vi "Teleop.vi"(10 "Match Info":T1={"Autonomous Elapsed Seconds"=0.0, "TeleOp Elapsed Seconds"=0.0, "Disabled Elapsed Seconds"=0.0, "Visited Autonomous"=FALSE, "Visited TeleOp"=FALSE, "Visited Disabled"=FALSE, "Autonomous Settings"={"Autonomous Style"=enum."Independent", "VI Refnum"=refnum}}, 11 "Call Context":T2) -> ()   [LabVIEW 2014]
doc: "This VI is called for each TeleOp packet received from the DS where the robot is not disabled. It is often used to read from the joysticks and update I/O or to update setpoints for timed control loops. It should complete and return within 20 milliseconds or it may miss DS packets."
uses:
  <vilib>/Rock Robotics/WPI/DriverStation/WPI_DriverStationDerivedRobotMode.ctl
  <vilib>/Rock Robotics/WPI/DriverStation/WPI_DriverStationMatch Info.ctl
  <vilib>/Rock Robotics/WPI/RobotDrive/WPI_RobotDriveGetSetRefNum.vi
  <vilib>/Rock Robotics/WPI/Joystick/WPI_JoystickGetSetRefNum.vi
  Robot Global Data.vi
  <vilib>/Rock Robotics/Network Tables/SD Write Boolean Array.vi
  <vilib>/Rock Robotics/Network Tables/SD Write Numeric Array.vi
  <vilib>/Rock Robotics/Network Tables/SD Read Boolean.vi
  <vilib>/Rock Robotics/Network Tables/SD Read Number.vi
  <vilib>/Rock Robotics/WPI/RobotDrive/WPI_RobotDriveArcadeDrive_Standard(NoSaturation).vi
panel:
  out "Sample Slider 0":dbl(slide) scale=0.0..5.0
  out "Sample Boolean 1":bool
  out "Sample Boolean 0":bool
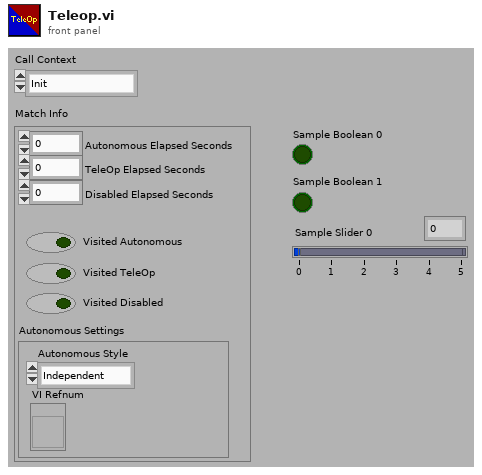
[diagram p1: front panel]
types:
  T1 = typedef "WPI_DriverStationMatch Info.ctl" = cluster{"Autonomous Elapsed Seconds":dbl, "TeleOp Elapsed Seconds":dbl, "Disabled Elapsed Seconds":dbl, "Visited Autonomous":bool, "Visited TeleOp":bool, "Visited Disabled":bool, "Autonomous Settings":cluster{"Autonomous Style":enum16{"Iterative", "Independent"}, "VI Refnum":refnum<vi>}}
  T2 = typedef "WPI_DriverStationDerivedRobotMode.ctl" = enum16{"Init", "Execute", "Stop"}
  T3 = typedef "WPI_RobotDriveDevRef.ctl" = cluster{"DevStatus":errorcluster, "Motors[]":T4[], "Square Inputs":bool, "Max Output":dbl}
  T4 = typedef "WPI_MotorControlDeviceRef.ctl" = cluster{"DeviceStatus":errorcluster, "Type":T5, "PWM":cluster{"Controller":T6, "PWM Channel":T7, "DeadBand":T8}, "CAN":cluster{"Device Number":u8, "Control Mode":T9, "Semaphore":T10, "Max Vout":dbl, "TalonSRX Control Mode":T11}, "Invert":bool, "TransformRef":T12, "InvTransformRef":T12}
  T5 = typedef "WPI_MotorControlType.ctl" = enum16{"PWM", "CAN", "CANTalonSRX"}
  T6 = typedef "FPGA_TypedefDigitalModule.ctl" = enum16{"Controller 1"}
  T7 = typedef "FPGA_DIOPWMChannel.ctl" = enum8{"PWM 0", "PWM 1", "PWM 2", "PWM 3", "PWM 4", "PWM 5", "PWM 6", "PWM 7", "PWM 8", "PWM 9", "PWM MXP 0", "PWM MXP 1", "PWM MXP 2", "PWM MXP 3", "PWM MXP 4", "PWM MXP 5", "PWM MXP 6", "PWM MXP 7", "PWM MXP 8", "PWM MXP 9", "Invalid"}
  T8 = typedef "WPI_PWMDeadband.ctl" = cluster{"Name":string, "maxPositivePwm":i32, "minPositivePwm":i32, "centerPwm":i32, "maxNegativePwm":i32, "minNegativePwm":i32, "angularRange":u16}
  T9 = typedef "WPI_CANJaguar_ControlMode.ctl" = enum8{"Percent VBus", "Current", "Speed", "Position", "Voltage"}
  T10 = typedef "Semaphore RefNum" = refnum<k1>
  T11 = typedef "WPI_CANTalonSRX_APIControlMode.ctl" = enum8{"Percent VBus", "Speed", "Position", "Slave", "Unchanged / Invalid"}
  T12 = typedef "WPI_PWMTransform_ConPane.ctl" = refnum<vi>
  T13 = typedef "WPI_JoystickDevRef.ctl" = cluster{"Device":T14}
  T14 = typedef "WPI_JoystickDeviceEnum.ctl" = enum16{"USB 0", "USB 1", "USB 2", "USB 3", "USB 4", "USB 5"}
  T15 = cluster{"Buttons[0]":bool, "Buttons[1]":bool, "Buttons[2]":bool, "Buttons[3]":bool, "Buttons[4]":bool, "Buttons[5]":bool, "Buttons[6]":bool, "Buttons[7]":bool, "Buttons[8]":bool}
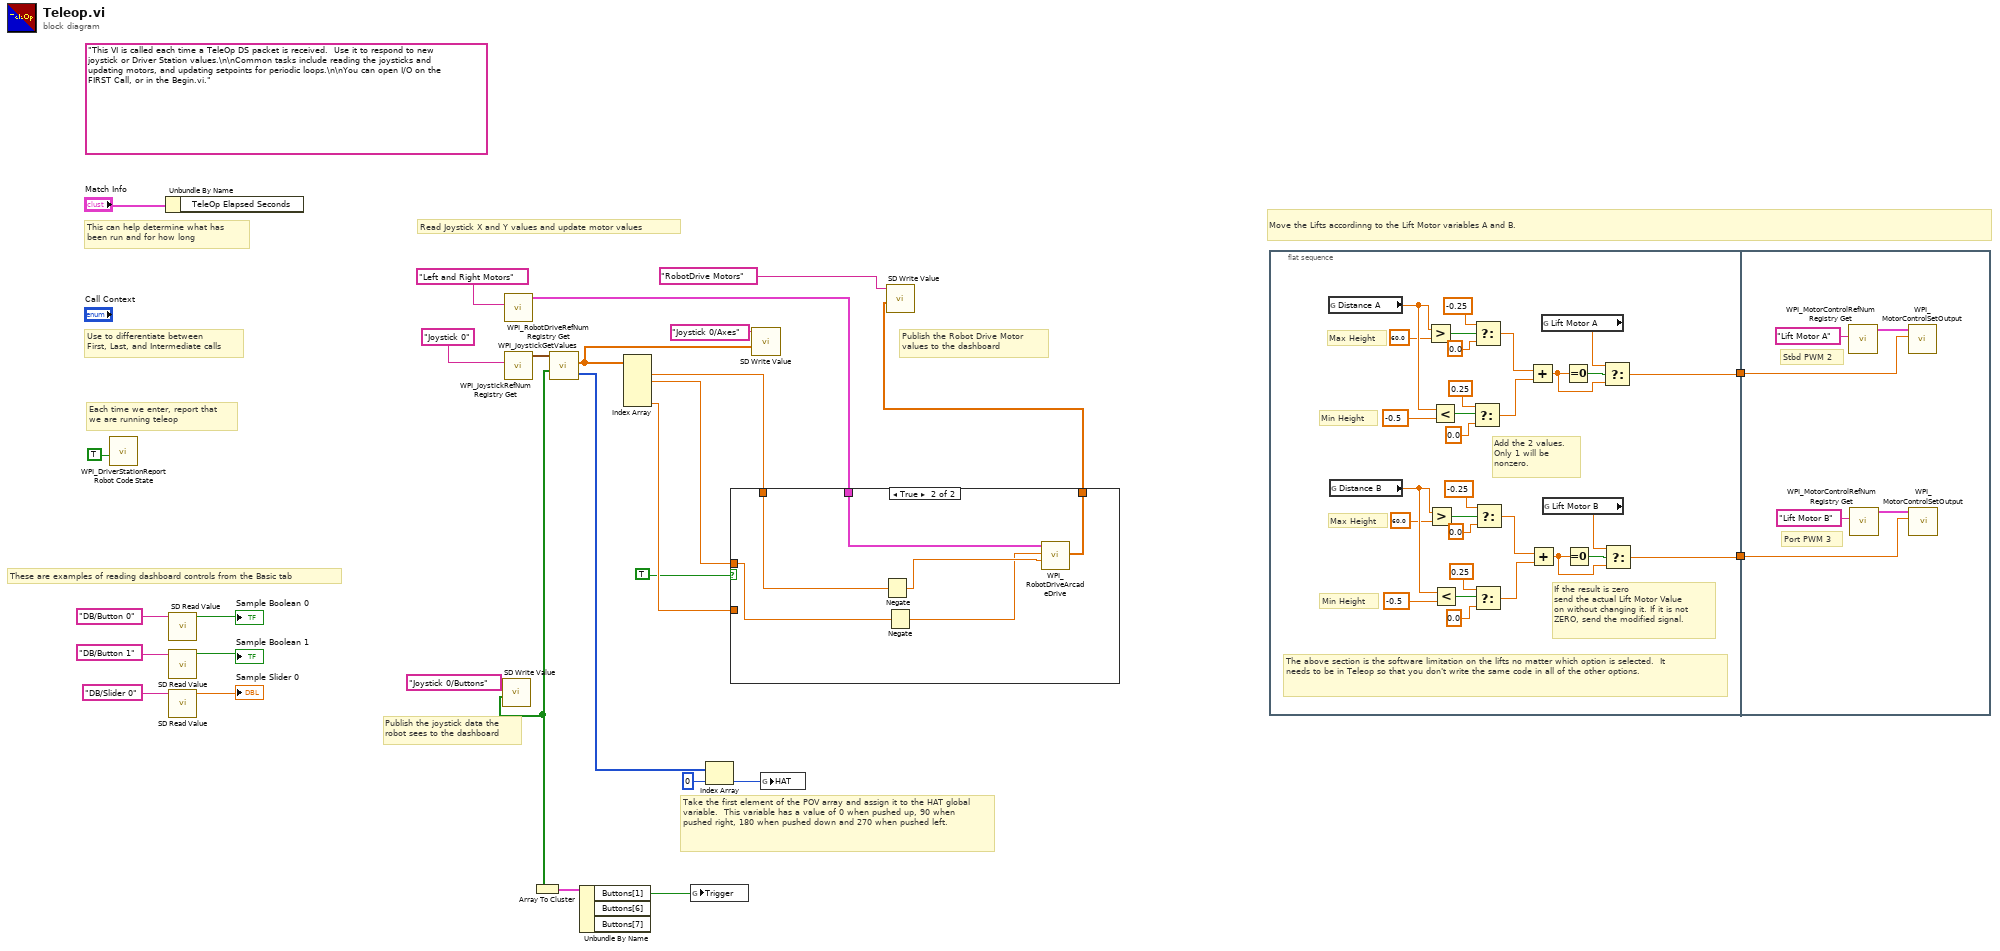
[diagram p0: block diagram]
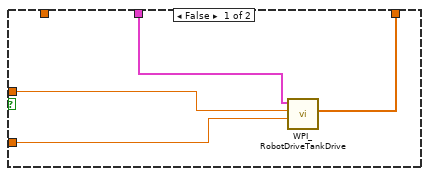
[diagram p2: hidden frame]
diagram:
  (unwired) "This VI is called each time a TeleOp DS packet is received.  Use it to respond to new joystick or Driver Station values.\n\nCommon tasks include reading the joysticks and updating motors, and updating setpoints for periodic loops.\n\nYou can open I/O on the FIRST Call, or in the Begin.vi."
  # "Move the Lifts accordinng to the Lift Motor variables A and B."
  # "Take the first element of the POV array and assign it to the HAT global variable.  This variable has a value of 0 when pushed up, 90 when pushed right, 180 when pushed down and 270 when pushed left."
  # "These are examples of reading dashboard controls from the Basic tab"
  # "Publish the Robot Drive Motor\nvalues to the dashboard"
  # "Publish the joystick data the\nrobot sees to the dashboard"
  # "Each time we enter, report that\nwe are running teleop"
  # "Use to differentiate between\nFirst, Last, and Intermediate calls"
  # "This can help determine what has\nbeen run and for how long"
  # "Read Joystick X and Y values and update motor values"
  n1 = call <vilib>:"WPI_DriverStationReport Robot Code State.vi"("TeleOp"=TRUE ("Autonomous")) -> ()  [unwired: 10 in, 1 out]
  n2 = Unbundle By Name("Match Info") -> ()  [unwired: 1 out]
  n3 = call-poly <vilib>:"SD Read Value.vi"("Name"="DB/Button 0" ("refnum name")) -> ("Boolean"=→"Sample Boolean 0":bool)  [unwired: 8 in, 2 out]
  n4 = call-poly <vilib>:"SD Read Value.vi"("Name"="DB/Button 1" ("refnum name")) -> ("Boolean"=→"Sample Boolean 1":bool)  [unwired: 8 in, 2 out]
  n5 = call-poly <vilib>:"SD Read Value.vi"("Name"="DB/Slider 0" ("refnum name")) -> ("Numeric"=→"Sample Slider 0":dbl)  [unwired: 8 in, 2 out]
  n6 = call <vilib>:"WPI_RobotDriveRefNum Registry Get.vi"("refnum name"="Left and Right Motors") -> ("RobotDriveDevRef"=w14:T3)  [unwired: 1 in, 9 out]
  n7 = call <vilib>:"WPI_JoystickRefNum Registry Get.vi"("refnum name"="Joystick 0") -> ("JoystickDevRef"=w26:T13)  [unwired: 1 in, 9 out]
  n8 = call <vilib>:"WPI_JoystickGetValues.vi"("JoystickDevRef"=w26) -> ("Buttons"=w13:bool[], "Axes"=w8:dbl[], "POVs"=w6:i16[])  [unwired: 6 in, 2 out]
  n9 = call-poly <vilib>:"SD Write Value.vi"("Boolean Array"=w13, "Name"="Joystick 0/Buttons") -> ()  [unwired: 8 in, 2 out]
  n10 = Array To Cluster(array=w13) -> (cluster=w12:T15)
  n11 = Unbundle By Name(w12) -> ("Buttons[1]"=w7:bool)  [unwired: 2 out]
  n12 = Index Array(array=w8) -> (element #1=w11:dbl, element #2=w10:dbl, element #5=w9:dbl)  [unwired: 5 in, 2 out]
  n13 = global write "Robot Global Data.vi" "Trigger"(w7) -> ()
  n14 = Index Array(array=w6, index=0) -> (element=w4:i16)
  n15 = case shown="True" TRUE {
    tunnel: [w33 w39] -> w15
    tunnel: w14 -> [w32 w38]
    tunnel: w11 -> [_ w37]
    tunnel: w10 -> [w31 w35]
    tunnel: w9 -> [w30 _]
    frame False {
      n16 = call <vilib>:"WPI_RobotDriveTankDrive.vi"("Right axis value"=w30, "Left axis value"=w31, "RobotDriveDevRef"=w32) -> ("Motor Values"=w33:dbl[])  [unwired: 6 in, 2 out]
    }
    frame True {
      n17 = Negate(x=w37) -> (-x=w36:dbl)
      n18 = Negate(x=w35) -> (-x=w34:dbl)
      n19 = call-poly <vilib>:"WPI_RobotDriveArcadeDrive.vi"("Y axis value"=w36, "X axis value"=w34, "RobotDriveDevRef"=w38) -> ("Motor Values"=w39:dbl[])  [unwired: 6 in, 2 out]
    }
  }
  n20 = call-poly <vilib>:"SD Write Value.vi"("Numeric Array"=w8, "Name"="Joystick 0/Axes") -> ()  [unwired: 8 in, 2 out]
  n21 = global write "Robot Global Data.vi" "HAT"(w4) -> ()
  n22 = call-poly <vilib>:"SD Write Value.vi"("Numeric Array"=w15, "Name"="RobotDrive Motors") -> ()  [unwired: 8 in, 2 out]
  n23 = flat-sequence {
    tunnel: [w41] -> w2
    tunnel: [w40] -> w1
    tunnel: w2 -> [w71]
    tunnel: w1 -> [w70]
    frame #0 {
      # "If the result is zero\nsend the actual Lift Motor Value\non without changing it. If it is not\nZERO, send the modified signal."
      # "Min Height"
      # "Max Height"
      # "Min Height"
      # "Max Height"
      # "The above section is the software limitation on the lifts no matter which option is selected.  It needs to be in Teleop so that you don't write the same code in all of the other options."
      # "Add the 2 values.  Only 1 will be nonzero."
      n24 = global read "Robot Global Data.vi" "Distance A"() -> (w61:dbl)
      n25 = global read "Robot Global Data.vi" "Distance B"() -> (w47:dbl)
      n26 = Greater?(x=w61, y=60.0) -> (0:w60:bool)
      n27 = Greater?(x=w47, y=60.0) -> (0:w46:bool)
      n28 = Less?(x=w61, y=-0.5) -> (x < y?=w63:bool)
      n29 = Less?(x=w47, y=-0.5) -> (x < y?=w49:bool)
      n30 = Select(t=0.25, s=w63, f=0.0) -> (s? t:f=w69:dbl)
      n31 = Select(t=-0.25, s=w60, f=0.0) -> (s? t:f=w68:dbl)
      n32 = Select(t=0.25, s=w49, f=0.0) -> (s? t:f=w55:dbl)
      n33 = Select(t=-0.25, s=w46, f=0.0) -> (s? t:f=w54:dbl)
      n34 = Add(x=w68, y=w69) -> (x+y=w56:dbl)
      n35 = Add(x=w54, y=w55) -> (x+y=w42:dbl)
      n36 = global read "Robot Global Data.vi" "Lift Motor A"() -> (w57:dbl)
      n37 = global read "Robot Global Data.vi" "Lift Motor B"() -> (w43:dbl)
      n38 = Equal To 0?(x=w56) -> (x = 0?=w58:bool)
      n39 = Equal To 0?(x=w42) -> (x = 0?=w44:bool)
      n40 = Select(t=w57, s=w58, f=w56) -> (s? t:f=w40:dbl)
      n41 = Select(t=w43, s=w44, f=w42) -> (s? t:f=w41:dbl)
    }
    frame #1 {
      # "Stbd PWM 2"
      # "Port PWM 3"
      n42 = call <vilib>:"WPI_MotorControlRefNum Registry Get.vi"("refnum name"="Lift Motor A") -> ("MotorControlDevRef"=w73:T4)  [unwired: 9 in, 1 out]
      n43 = call <vilib>:"WPI_MotorControlRefNum Registry Get.vi"("refnum name"="Lift Motor B") -> ("MotorControlDevRef"=w75:T4)  [unwired: 9 in, 1 out]
      n44 = call <vilib>:"WPI_MotorControlSetOutput.vi"("Output"=w70, "MotorControlDevRef"=w73) -> ()  [unwired: 7 in, 3 out]
      n45 = call <vilib>:"WPI_MotorControlSetOutput.vi"("Output"=w71, "MotorControlDevRef"=w75) -> ()  [unwired: 7 in, 3 out]
    }
  }
